vi "Core_Stop.vi"(8 "error in (no error)":errorcluster, 11 "HSMS Class in":refnum<class "HSMS Class.lvclass">) -> (0 "error out":errorcluster, 3 "HSMS Class out":refnum<class "HSMS Class.lvclass">)   [LabVIEW 2020, in "SECS Communication.lvlib" / "HSMS Class.lvclass"]
uses:
  HSMS Class.lvclass
  HSMS State.ctl
  Notifier Type.ctl
  HSMS Class.lvclass/HSMS Class.ctl
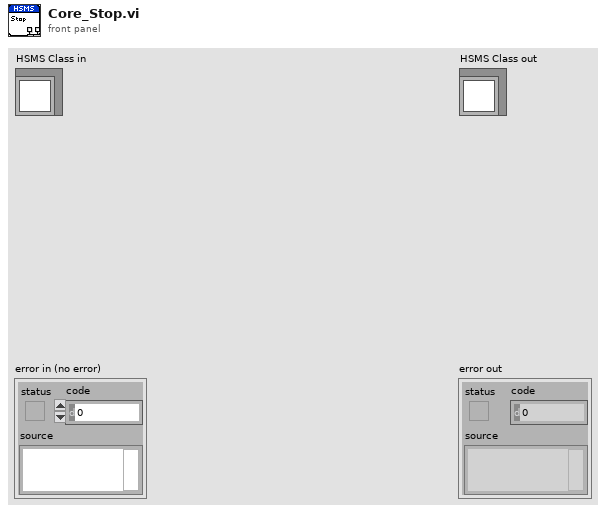
[diagram p1: front panel]
types:
  T1 = typedef "SECS Communication.lvlib/HSMS Class.lvclass/Notifier Type.ctl" = enum16{"TCPIP Connect", "TCPIP Disconnect", "Receive Message", "Send Message", "T3 Timeout", "T6 Timeout", "T7 Timeout", "Error", "Stop"}
  T2 = typedef "SECS Communication.lvlib/HSMS Class.lvclass/HSMS State.ctl" = enum16{"[TCP/IP]Not Connect", "[HSMS]Not Selected", "[HSMS]Selected", "Stop"}
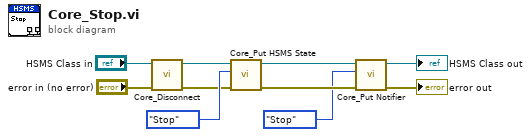
[diagram p0: block diagram]
diagram:
  n1 = call "Core_Disconnect.vi"("error in (no error)"="error in (no error)", "HSMS Class in"="HSMS Class in") -> ("error out"=w3:errorcluster, "HSMS Class out"=w4:refnum<class "HSMS Class.lvclass">)  [unwired: 8 in]
  n2 = call "Core_Put HSMS State.vi"("error in (no error)"=w3, "HSMS State"=HSMS_State."Stop", "HSMS Class in"=w4) -> ("error out"=w9:errorcluster, "HSMS Class out"=w7:refnum<class "HSMS Class.lvclass">)  [unwired: 7 in]
  n3 = call "Core_Put Notifier.vi"("error in (no error)"=w9, "Notifier Type"=Notifier_Type."Stop", "HSMS Class in"=w7) -> ("error out"=→"error out":errorcluster, "HSMS Class out"=→"HSMS Class out":refnum<class "HSMS Class.lvclass">)  [unwired: 7 in]
